vi "LV SciSDK INIT REGISTER FILE.vi"(9 "Handle In":T1, 11 "Register file name":string) -> (1 "Handle Out":T1, 2 "Register File Handle Out":T2)   [LabVIEW 2021, in "SciSDK_Labview.lvlib"]
uses:
  SciSDK_Labview.lvlib
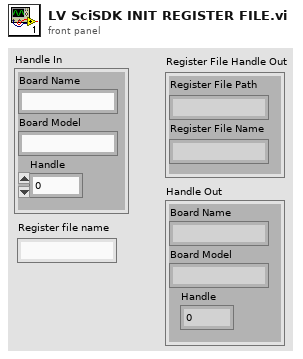
[diagram p1: front panel]
types:
  T1 = cluster{"Board Name":string, "Board Model":string, "Handle":u64}
  T2 = cluster{"Register File Path":string, "Register File Name":string}
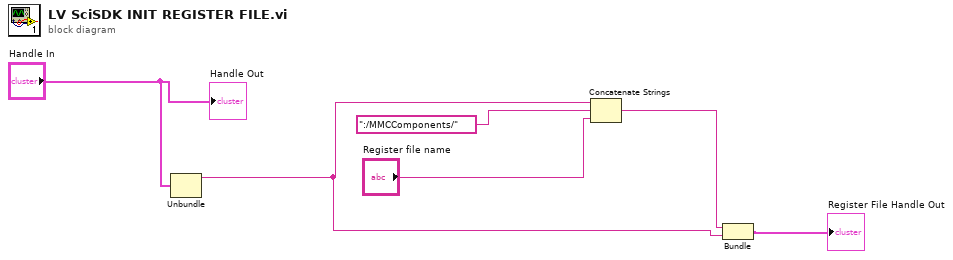
[diagram p0: block diagram]
diagram:
  n1 = Unbundle("Handle In") -> ("Board Name"=w1:string)  [unwired: 2 out]
  n2 = Concatenate Strings(w1, ":/MMCComponents/" ("string"), "Register file name") -> (w2:string)
  n3 = Bundle(w2, "Board Name"=w1) -> (→"Register File Handle Out":cluster{string, "Board Name":string})  [unwired: 1 in]
  "Handle Out" <- "Handle In"
